vi "Unsupported Data Type Error.vi"(8 "error in (no error)":errorcluster, 11 "Type Enum":T1) -> (0 "error out":errorcluster)   [LabVIEW 2013, in "JKI JSON Serialization.lvlib" / "JSON Serializer.lvclass"]
uses:
  JSON Serializer.lvclass
  <vilib>/Utility/VariantDataType/Type.ctl
  <vilib>/Utility/VariantDataType/VariantType.lvlib
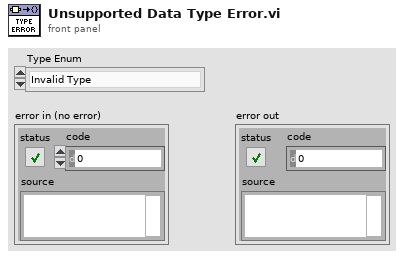
[diagram p1: front panel]
types:
  T1 = typedef "VariantType.lvlib/Type.ctl" = enum8{"Invalid Type", "Void", "I8", "I16", "I32", "I64", "U8", "U16", "U32", "U64", "Single Float", "Double Float", "Extended Float", "Single Complex", "Double Complex", "Extended Complex", "Enum U8", "Enum U16", "Enum U32", "Enum U64", "Single Float With Unit", "Double Float With Unit", "Extended Float With Unit", "Single Complex with Unit", "Double Complex with Unit", "Extended Complex with Unit", "Boolean", "String", "Path", "Picture", "Tag", "Array", "Cluster", "Variant", "LV Variant", "Waveform", "Timestamp", "Digital Waveform", "Digital Data", "ExpressData", "Refnum", "External Data", "VI", "Poly VI", "LabVIEW Class Instance", "Fixed Point"}
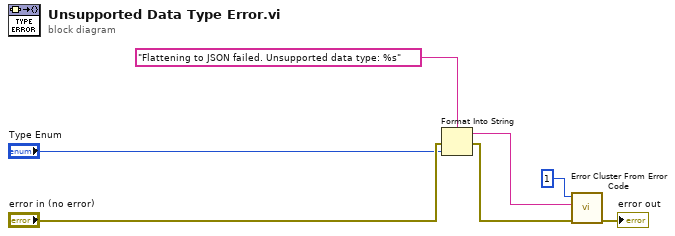
[diagram p0: block diagram]
diagram:
  n1 = Format Into String(format string="Flattening to JSON failed. Unsupported data type: %s" ("error message (\"\")"), error in="error in (no error)", "Type Enum") -> (resulting string=w5:string, error out=w7:errorcluster)  [unwired: 1 in]
  n2 = call <vilib>:"Error Cluster From Error Code.vi"("error in (no error)"=w7, "error message (\"\")"=w5, "error code (0)"=1) -> ("error out"=→"error out":errorcluster)  [unwired: 6 in]
